vi "Memory.Pointer.Move Block (unsafe).vi"(0 "src Pointer in":refnum<class "Memory.Pointer.lvclass">, 1 "length":i64 format="%d bytes", 5 "dst Pointer in":refnum<class "Memory.Pointer.lvclass">, 7 "src offset (0)":i64 format="%d bytes", 9 "dst offset (0)":i64 format="%d bytes", 11 "error in (no error)":errorcluster) -> (4 "src Pointer out":refnum<class "Memory.Pointer.lvclass">, 6 "dst Pointer out":refnum<class "Memory.Pointer.lvclass">, 15 "error out":errorcluster)   [LabVIEW 2016, in "LabVIEW Memory Manager.lvlib" / "Memory.Pointer.lvclass"]
uses:
  Memory.Pointer.lvclass
  Memory.Pointer.lvclass/Memory.Pointer.ctl
  Accessors/Memory.Pointer.Get Address.vi
  VIs/Memory.Truncate I64 to I32.vi
  LabVIEW Memory Manager.lvlib
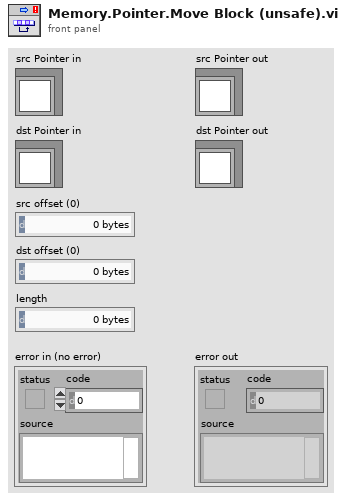
[diagram p1: front panel]
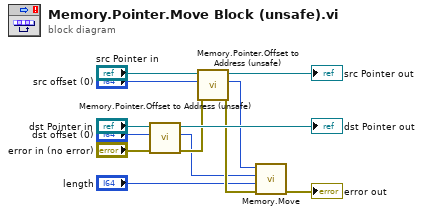
[diagram p0: block diagram]
diagram:
  n1 = call "Memory.Pointer.Offset to Address (unsafe).vi"("error in (no error)"="error in (no error)", "offset"="dst offset (0)", "Pointer in"="dst Pointer in") -> ("error out"=w11:errorcluster, "address"=w2:u64, "Pointer out"=→"dst Pointer out":refnum<class "Memory.Pointer.lvclass">)  [unwired: 6 in]
  n2 = call "Memory.Pointer.Offset to Address (unsafe).vi"("error in (no error)"=w11, "offset"="src offset (0)", "Pointer in"="src Pointer in") -> ("error out"=w5:errorcluster, "address"=w3:u64, "Pointer out"=→"src Pointer out":refnum<class "Memory.Pointer.lvclass">)  [unwired: 6 in]
  n3 = call "Memory.Move.vi"("error in (no error)"=w5, "size"="length", "dst address"=w2, "src address"=w3) -> ("error out"=→"error out":errorcluster)  [unwired: 7 in]
